vi "配置文件保存.vi"   [LabVIEW 2016, in "斯坦道多参数.lvlib"]
uses:
  <vilib>/Utility/config.llb/NI_LVConfig.lvlib
types:
  T1 = typedef "NI_LVConfig.lvlib/Config Data RefNum.ctl" = refnum<k1>
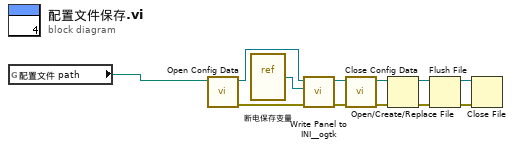
[diagram p0: block diagram]
diagram:
  n1 = global read "多参数全局变量.vi" "配置文件 path"() -> (w1:path)
  n2 = call <vilib>:"Open Config Data.vi"("configuration file path"=w1) -> ("error out"=w11:errorcluster, "refnum"=w12:T1)  [unwired: 8 in, 1 out]
  n3 = vi-ref "断电保存变量.vi"() -> (w8:refnum<vi>)
  n4 = call <userlib>:"Write Panel to INI__ogtk.vi"("error in (no error)"=w11, "VI ref"=w8, "refnum"=w12) -> ("error out"=w9:errorcluster, "refnum out"=w10:T1)  [unwired: 7 in]
  n5 = call <vilib>:"Close Config Data.vi"("error in (no error)"=w9, "refnum"=w10) -> ("error out"=w4:errorcluster, "file path"=w5:path)  [unwired: 8 in]
  n6 = Open/Create/Replace File(file path (use dialog)=w5, error in=w4) -> (refnum out=w6:refnum<file>, error out=w7:errorcluster)  [unwired: 4 in, 1 out]
  n7 = Flush File(refnum=w6, error in=w7) -> (refnum out=w2:refnum<file>, error out=w3:errorcluster)
  n8 = Close File(refnum=w2, error in=w3) -> ()  [unwired: 2 out]
